vi "String_in_Reference.vi"(13 "String":string) -> (18 "String Out":string)   [LabVIEW 2016]
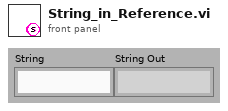
[diagram p1: front panel]
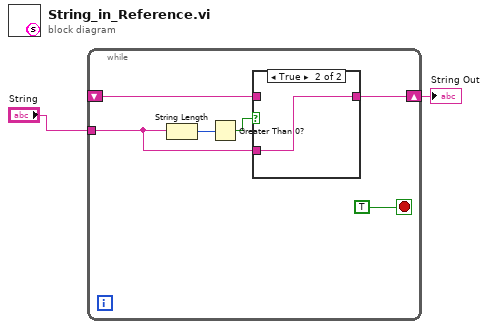
[diagram p0: block diagram]
diagram:
  n1 = while {
    shift-right: [w5] -> w1
    shift-left: _ -> [w4]
    tunnel: "String" -> [w3]
    stop <- TRUE stop-if-true
    n2 = String Length(string=w3) -> (length=w7:i32)
    n3 = Greater Than 0?(x=w7) -> (x > 0?=w6:bool)
    n4 = case shown="True" w6 {
      tunnel: [w9 w10] -> w5
      tunnel: w4 -> [w9 _]
      tunnel: w3 -> [_ w10]
      frame False {
      }
      frame True {
      }
    }
  }
  "String Out" <- w1
